vi "new AND Filter.vi"(5 "a":refnum<class "Filter.lvclass">, 9 "b":refnum<class "Filter.lvclass">) -> (8 "a and b":refnum<class "Filter.lvclass">)   [LabVIEW 2016, in "FPGA Resource Manager.lvlib" / "AND Filter.lvclass"]
uses:
  AND Filter.lvclass
  Filter Parent/Filter.lvclass
  C:/github/VeriStand-FPGA-Resource-Manager/Source/Client/Test CD/FPGA RM Test Client/Source/System Explorer/Filters/Filter Parent/Filter.lvclass
  AND Filter.lvclass/AND Filter.ctl
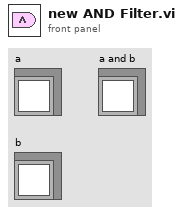
[diagram p1: front panel]
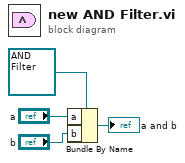
[diagram p0: block diagram]
diagram:
  n1 = Bundle By Name(cluster=refnum<class "AND Filter.lvclass"> refnum ("And Filter in"), "a"="a", "b"="b") -> (→"a and b":refnum<class "AND Filter.lvclass">)
